vi "Create RDMA Error.vi"(9 "source vi name":string, 11 "error":T1) -> (1 "offset":i32, 3 "error out":errorcluster)   [LabVIEW 2020, in "RDMA.lvlib" / "RDMA Transceiver.lvclass"]
uses:
  RDMA Transceiver.lvclass
  Library Name.vi
  <vilib>/NI/Memory Manager/Static Errors.lvlib
  <vilib>/NI/Memory Manager/VIs/New Error Cluster (512B).vi
  Errors.ctl
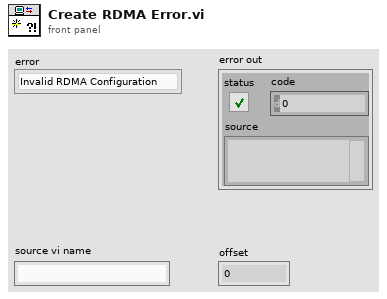
[diagram p1: front panel]
types:
  T1 = typedef "RDMA.lvlib/RDMA Transceiver.lvclass/Errors.ctl" = enum16{"Invalid RDMA Configuration", "Too Many Transfers", "Size Mismatch", "Unknown Setting"}
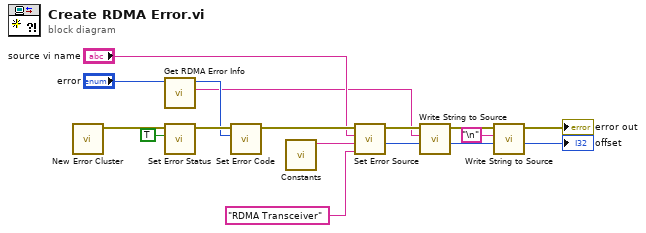
[diagram p0: block diagram]
diagram:
  n1 = call-poly <vilib>:"New Error Cluster.vi"() -> ("error out"=w16:errorcluster)  [unwired: 10 in, 1 out]
  n2 = call "Get RDMA Error Info.vi"("error"="error") -> ("description"=w7:string, "code"=w10:i32)  [unwired: 9 in]
  n3 = call <vilib>:"Set Error Status.vi"("status (T)"=TRUE, "error in"=w16) -> ("error out"=w14:errorcluster)  [unwired: 9 in]
  n4 = call <vilib>:"Set Error Code.vi"("code"=w10, "error in"=w14) -> ("error out"=w13:errorcluster)  [unwired: 9 in]
  n5 = call-poly "Constants.vi"() -> ("library name"=w11:string)  [unwired: 11 in]
  n6 = call <vilib>:"Set Error Source.vi"("class name (\"\")"="RDMA Transceiver" ("class name (\"\")"), "library name (\"\")"=w11, "vi name"="source vi name", "error in"=w13) -> ("initial offset"=w8:i32, "error out"=w9:errorcluster)  [unwired: 6 in]
  n7 = call <vilib>:"Write String to Source.vi"("offset"=w8, "string"=w7, "error in"=w9) -> ("new offset"=w5:i32, "error out"=w6:errorcluster)  [unwired: 7 in]
  n8 = call <vilib>:"Write String to Source.vi"("offset"=w5, "string"="\n", "error in"=w6) -> ("new offset"=→"offset":i32, "error out"=→"error out":errorcluster)  [unwired: 7 in]
